vi "Get Set Warning.vi"(8 "Error In":errorcluster, 10 "UIP":refnum<class "UIP.lvclass">, 11 "Label.Text":string) -> (0 "Error Out":errorcluster)   [LabVIEW 2015, in "UIM.lvclass"]
uses:
  UIM.lvclass
  UIP/UIP.lvclass
  <vilib>/Utility/error.llb/Error Cluster From Error Code.vi
  <vilib>/ErrorRing/Error Ring.xnode
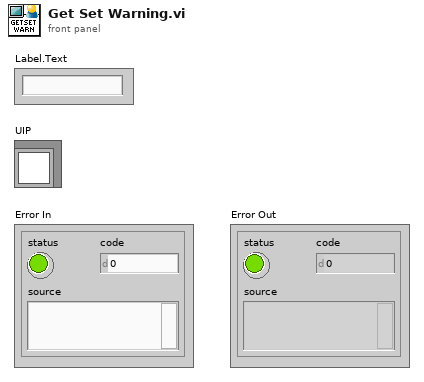
[diagram p1: front panel]
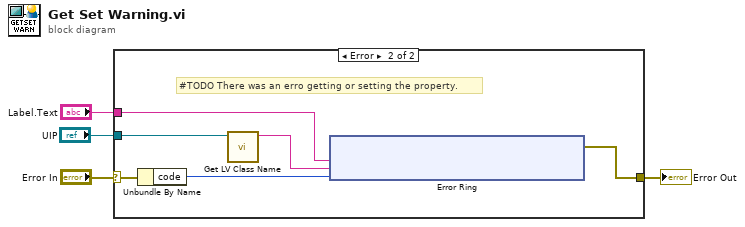
[diagram p0: block diagram]
diagram:
  n1 = case shown="Error" "Error In" {
    selector: "Error In" -> [w5 w11]
    tunnel: "Label.Text" -> [_ w9]
    tunnel: [w5 w6] -> w4
    tunnel: "UIP" -> [_ w10]
    frame No Error {
    }
    frame Error {
      # "#TODO There was an erro getting or setting the property."
      n2 = Unbundle By Name(w11) -> ("code"=w7:i32)
      n3 = call <vilib>:"Get LV Class Name.vi"("object"=w10) -> ("class name"=w8:string)  [unwired: 9 in, 1 out]
      n4 = xnode "Error Ring"("parameter 0"=w9, "parameter 1"=w8, "parameter 2"=w7) -> ("error out"=w6:errorcluster)
    }
  }
  "Error Out" <- w4
